vi "NewChicagoStyleVeggiePizza.vi"(8 "error in (no error)":errorcluster) -> (0 "error out":errorcluster, 3 "ChicagoStyleVeggiePizza":refnum<class "ChicagoStyleVeggiePizza.lvclass">)   [LabVIEW 2020, in "FactoryMethod.lvlib" / "PizzaFactoryMethod.lvlib" / "ChicagoStyleVeggiePizza.lvclass"]
uses:
  ChicagoStyleVeggiePizza.lvclass
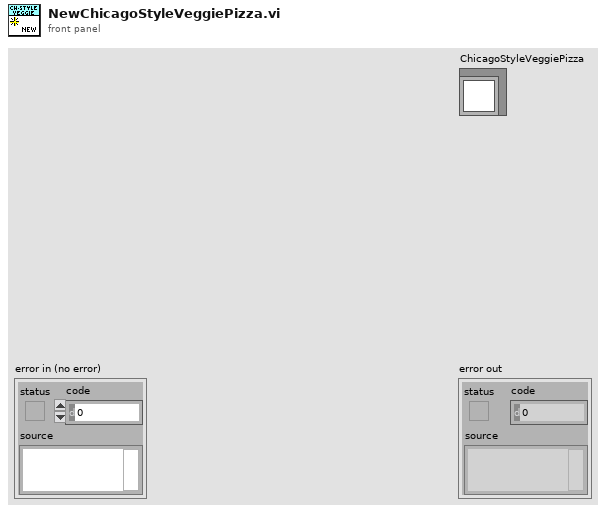
[diagram p1: front panel]
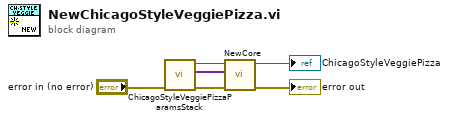
[diagram p0: block diagram]
diagram:
  n1 = call "ChicagoStyleVeggiePizzaParamsStack.vi"("error iN"="error in (no error)") -> ("error out"=w6:errorcluster, "HierarchyParams"=w5:variant[], "ChicagoStyleVeggiePizza"=w1:refnum<class "ChicagoStyleVeggiePizza.lvclass">)  [unwired: 8 in]
  n2 = call-dynamic "NewCore.vi"("error in (no error)"=w6, "ParamsArray"=w5, "ChicagoStyleVeggiePizza"=w1) -> ("error out"=→"error out":errorcluster, "ChicagoStyleVeggiePizza"=→"ChicagoStyleVeggiePizza":refnum<class "ChicagoStyleVeggiePizza.lvclass">)  [unwired: 7 in]
